vi "acq.Single.vi"(7 "DVR":T2, 8 "error in":errorcluster, 10 "image":refnum<queue>) -> (0 "error out":errorcluster, 2 "Image Out":T1, 4 "acq time":dbl)   [LabVIEW 2020]
uses:
  _controls/data.ref.ctl
  _controls/data.ctl
  _controls/state.ctl
  _controls/data.vars.ctl
  _controls/flip.ctl
  <vilib>/vision/Image Controls.llb/IMAQ Image.ctl
  camera/camera.lvclass
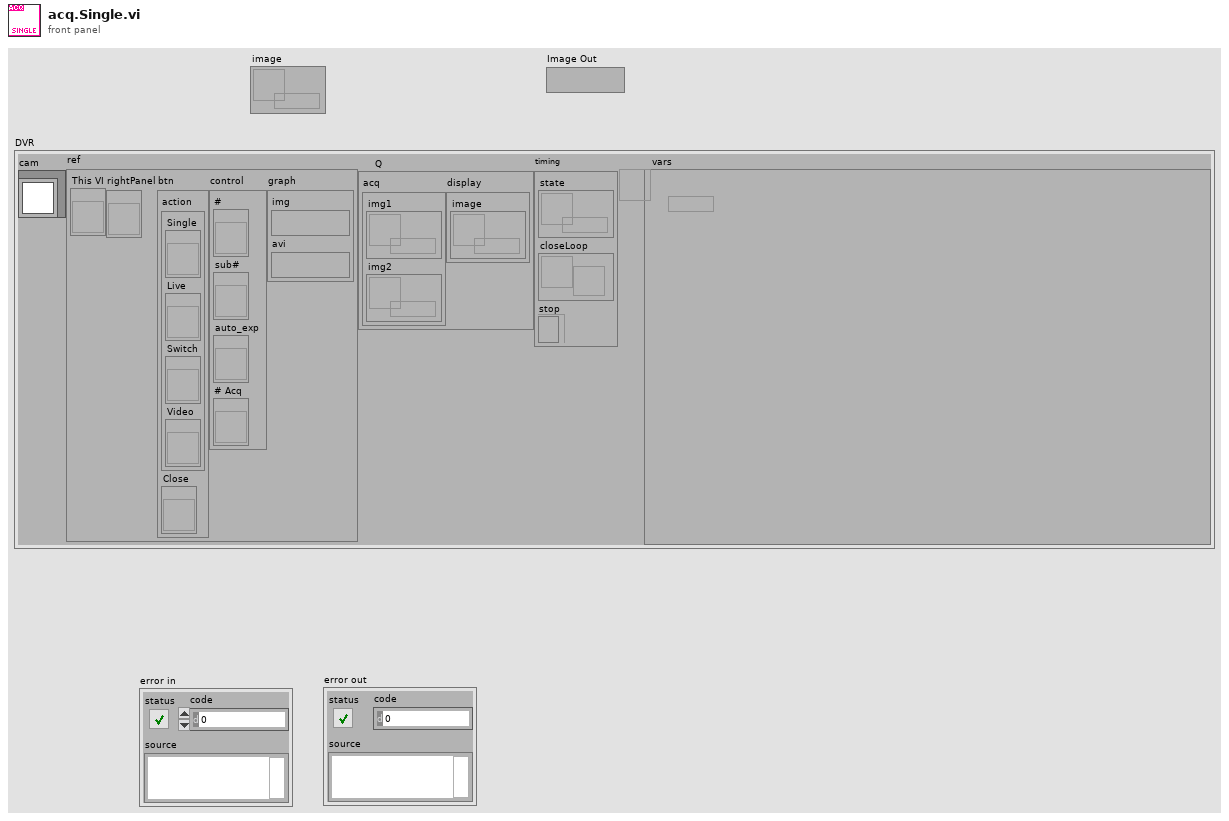
[diagram p1: front panel]
types:
  T1 = typedef "IMAQ Image.ctl" = refnum<image>
  T2 = typedef "data.ctl" = cluster{"cam":refnum<class "camera.lvclass">, "ref":T3, "Q":cluster{"acq":cluster{"img1":refnum<queue>, "img2":refnum<queue>}, "display":cluster{"image":refnum<queue>}}, "timing":cluster{"state":refnum<queue>, "closeLoop":refnum<notifier>, "stop":refnum<k4>}, "vars":refnum<data-value>}
  T3 = typedef "data.ref.ctl" = cluster{"This VI":refnum<vi>, "rightPanel":refnum<vi>, "btn":cluster{"action":cluster{"Single":refnum<vi>, "Live":refnum<vi>, "Switch":refnum<vi>, "Video":refnum<vi>}, "Close":refnum<vi>}, "control":cluster{"#":refnum<vi>, "sub#":refnum<vi>, "auto_exp":refnum<vi>, "# Acq":refnum<vi>}, "graph":cluster{"img":T1, "avi":T1}}
  T4 = typedef "data.vars.ctl" = cluster{"save":cluster{"base_folder":cluster{"Folder":path, "tif":bool, "jpg":bool}, "module":string, "#":u32, "sub#":u8, "save.op":enum16{"Full", "Light"}, "same?":bool, "Shift":enum16{"Single", "Leapfrog"}, "jpg?":bool, "flip":T5}, "acq":cluster{"# Acq":u16, "rotate":bool, "FPS":dbl}, "calib.manual":cluster{"BG":cluster{"Image":u16[][], "enabled?":bool}, "FF":cluster{"Image":u16[][], "enabled?":bool}}}
  T5 = typedef "flip.ctl" = cluster{"x":bool, "y":bool}
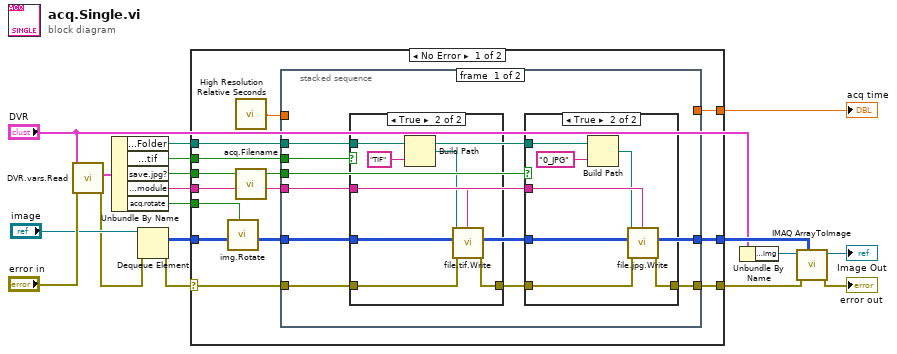
[diagram p0: block diagram]
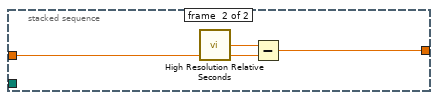
[diagram p4: hidden frame]
diagram:
  n1 = call "DVR.vars.Read.vi"("error in"="error in", "DVR.state"="DVR") -> ("error out"=w1:errorcluster, "vars"=w18:T4)  [unwired: 8 in]
  n2 = Unbundle By Name(w18) -> ("save.base_folder.Folder"=w17:path, "save.base_folder.tif"=w13:bool, "save.jpg?"=w16:bool, "save.module"=w14:string, "acq.rotate"=w11:bool)
  n3 = Dequeue Element(queue="image", error in (no error)=w1) -> (element=w4:u16[][], error out=w2:errorcluster)  [unwired: 1 in, 2 out]
  n4 = case shown="No Error" w2 {
    selector: w2 -> [w23 w59]
    tunnel: w17 -> [w30 _]
    tunnel: w16 -> [w26 _]
    tunnel: [w25 _] -> w15
    tunnel: [w22 w59] -> w9
    tunnel: [w24 _] -> w7
    tunnel: w14 -> [w29 _]
    tunnel: w13 -> [w28 _]
    tunnel: w11 -> [w21 _]
    tunnel: w4 -> [w20 _]
    frame No Error {
      n5 = call "img.Rotate.vi"("rotate"=w21, "image in"=w20) -> ("image out"=w19:u16[][])  [unwired: 9 in]
      n6 = call <vilib>:"High Resolution Relative Seconds.vi"() -> ("relative seconds"=w31:dbl)
      n7 = call "acq.Filename.vi"("module"=w29) -> ("filename"=w27:string)  [unwired: 10 in]
      n8 = stacked-sequence {
        tunnel: [w34 _] -> w22
        tunnel: w31 -> [_ w57]
        tunnel: [_ w56] -> w25
        tunnel: w23 -> [w33 _]
        tunnel: w30 -> [w38 _]
        tunnel: [w32 _] -> w24
        tunnel: w27 -> [w36 _]
        tunnel: w28 -> [w39 _]
        tunnel: w26 -> [w35 _]
        tunnel: w19 -> [w32 _]
        frame #0 {
          n9 = case shown="True" w39 {
            tunnel: w38 -> [_ w55]
            tunnel: w33 -> [w48 w54]
            tunnel: w36 -> [_ w53]
            tunnel: [w48 w52] -> w37
            tunnel: w32 -> [_ w49]
            frame False {
            }
            frame True {
              n10 = Build Path(base path=w55, name or relative path="TIF" ("filename")) -> (appended path=w50:path)
              n11 = call "file.tif.Write.vi"("name"=w53, "error in"=w54, "u16 pixmap"=w49, "path"=w50) -> ("error out"=w52:errorcluster)  [unwired: 7 in]
            }
          }
          n12 = case shown="True" w35 {
            tunnel: w38 -> [_ w47]
            tunnel: w37 -> [w40 w46]
            tunnel: w36 -> [_ w45]
            tunnel: [w40 w44] -> w34
            tunnel: w32 -> [_ w41]
            frame False {
            }
            frame True {
              n13 = Build Path(base path=w47, name or relative path="0_JPG" ("filename")) -> (appended path=w42:path)
              n14 = call "file.jpg.Write.vi"("name"=w45, "error in"=w46, "u16 pixmap"=w41, "path"=w42) -> ("error out"=w44:errorcluster)  [unwired: 7 in]
            }
          }
        }
        frame #1 {
          n15 = call <vilib>:"High Resolution Relative Seconds.vi"() -> ("relative seconds"=w58:dbl)
          n16 = Subtract(x=w58, y=w57) -> (x-y=w56:dbl)
        }
      }
    }
    frame Error {
    }
  }
  "acq time" <- w15
  n17 = Unbundle By Name("DVR") -> ("ref.graph.img"=w10:T1)
  n18 = call "IMAQ ArrayToImage"("Image Pixels (U16)"=w7, "error in (no error)"=w9, "Image"=w10) -> ("error out"=→"error out":errorcluster, "Image Out"=→"Image Out":T1)  [unwired: 7 in]
